vi "NI9252_CREATE_TASK.vi"() -> ()   [LabVIEW 2022 SP3]
uses:
  <vilib>/Analysis/baseanly.llb/Mean (DBL).vi
  <vilib>/express/express shared/transition.llb/Dynamic To Waveform Array.vi
  <vilib>/express/express signal manip/GetorSetDDTAttributes/Set DDT Attributes/SetT0.vi
  <vilib>/express/express signal manip/GetorSetDDTAttributes/Set DDT Attributes/sub Set StartTimeStamp.vi
  <vilib>/express/express shared/transition.llb/Waveform Array To Dynamic.vi
  <vilib>/express/express signal manip/GetorSetDDTAttributes/Set DDT Attributes/Set DDT Properties.xnode
  <vilib>/Analysis/NI_AALBase.lvlib
  <vilib>/express/express signal manip/GetorSetDDTAttributes/Set DDT Attributes/Set DDT Attributes.lvlib
panel:
  in  "Enable":bool=TRUE
  in  "number of samples":i32=60
  in  "rate":dbl=60.0
  out "Waveform Graph 2":dbl[](graph)
  out "Waveform Graph":dbl[](graph)
  out "Waveform Chart 2":dynamicdata(graph)
  out "Waveform Chart":dynamicdata(graph)
  out "Saving Data":bool
  out "Filename Out":path
  in  "Filename":path=path "C:/1. Rocket Research Project/CollectedData/Test_Firing/Constant Chamber Pressure/DataFileThrustWooden.lvm"
  in  "Signal Index 2":i32
  in  "Signal Index":i32
  in  "stop":bool
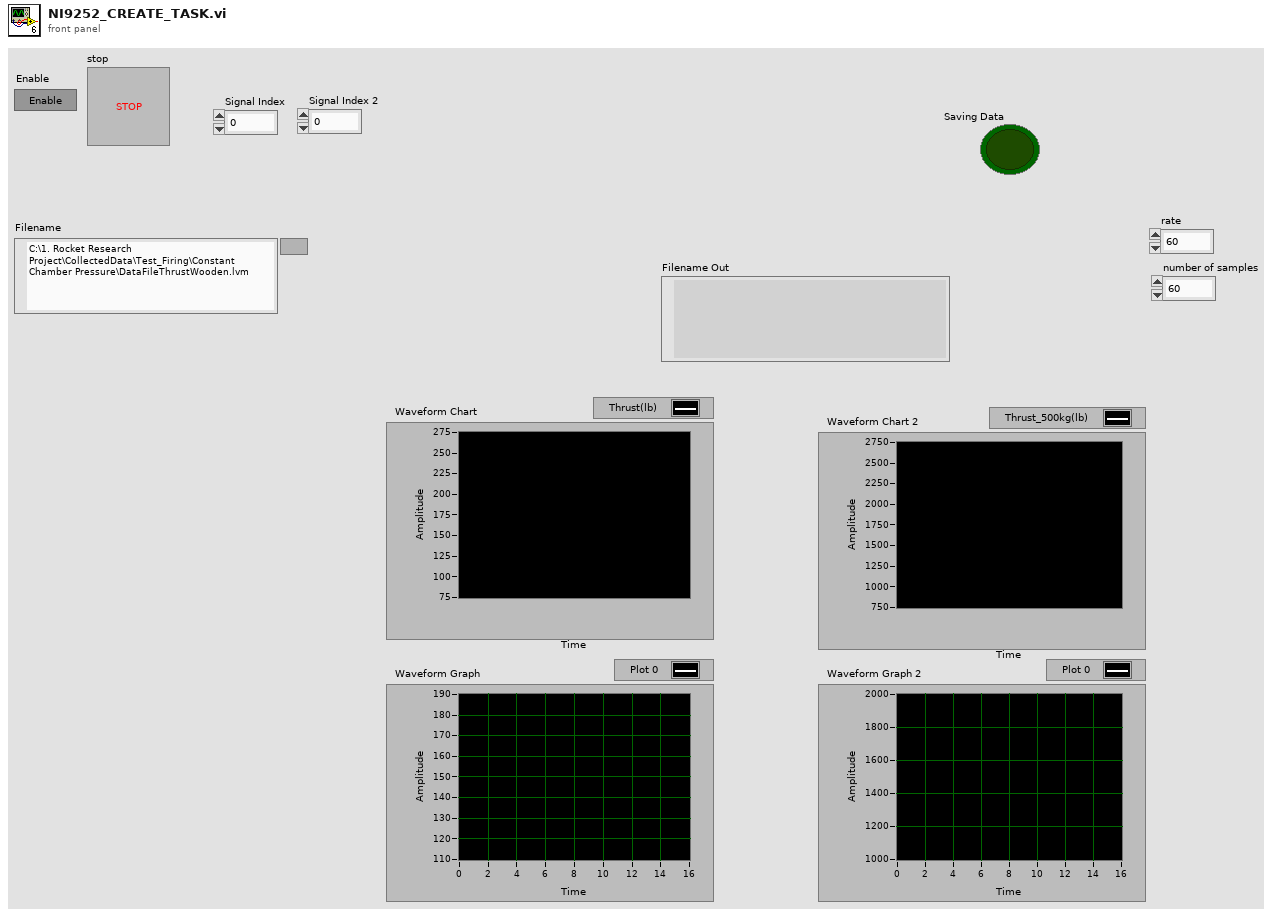
[diagram p1: front panel]
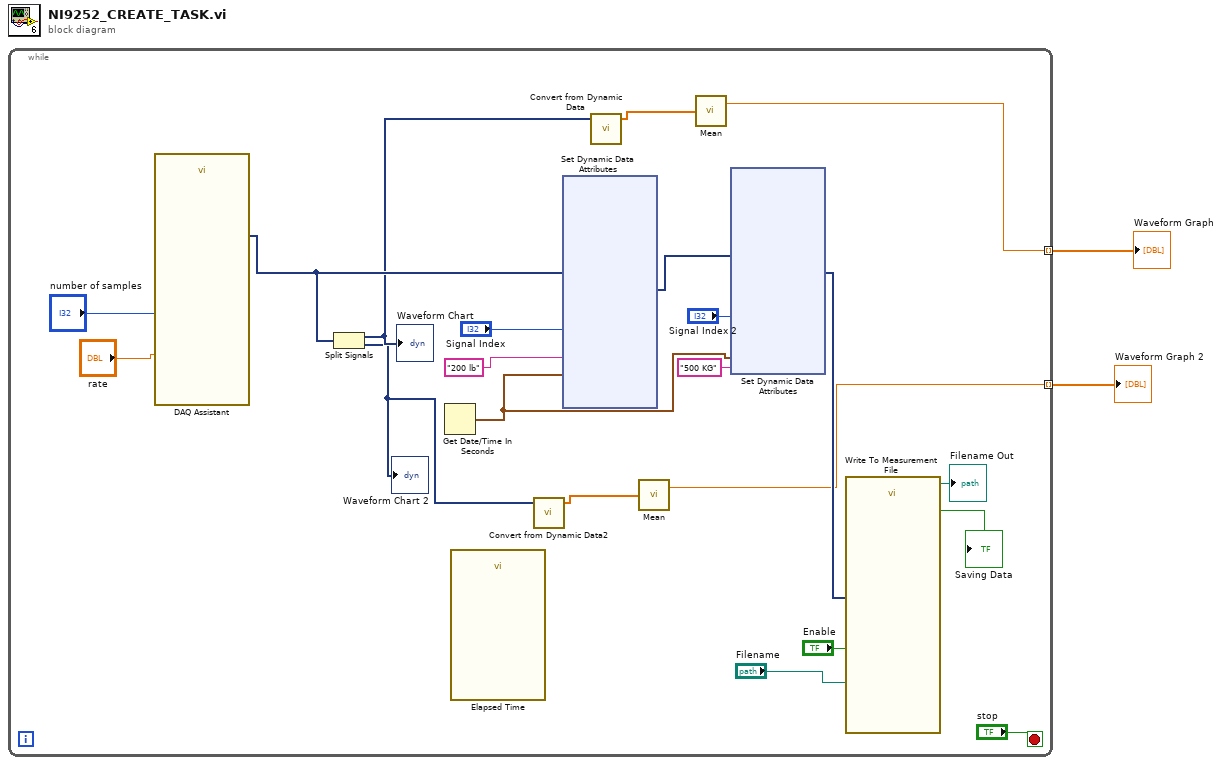
[diagram p0: block diagram]
diagram:
  n1 = while {
    tunnel: [w10] -> w2 mode=indexing
    tunnel: [w7] -> w1 mode=indexing
    stop <- "stop" stop-if-true
    n2 = call "DAQ Assistant"("rate"="rate", "number of samples"="number of samples") -> ("data"=w13:dynamicdata)  [unwired: 14 in, 3 out]
    n3 = Split Signals(w13) -> (w12:dynamicdata, w8:dynamicdata)  [unwired: 2 in]
    "Waveform Chart" <- w12
    "Waveform Chart 2" <- w8
    n4 = Get Date/Time In Seconds() -> (seconds since 1Jan1904=w4:timestamp)
    n5 = call "Elapsed Time"() -> ()  [unwired: 12 in, 8 out]
    n6 = call "Convert from Dynamic Data2"("Dynamic Data Type"=w8) -> ("Array"=w9:dbl[])  [unwired: 3 in]
    n7 = xnode "Set Dynamic Data Attributes"("Signals In"=w13, "Signal Index"="Signal Index", "Signal Name"="200 lb", "Start Timestamp"=w4) -> ("Signals Out"=w20:dynamicdata)  [unwired: 2 in, 1 out]
    n8 = call "Convert from Dynamic Data"("Dynamic Data Type"=w12) -> ("Array"=w11:dbl[])  [unwired: 3 in]
    n9 = call-poly <vilib>:"Mean.vi"("X"=w9) -> ("mean"=w7:dbl)  [unwired: 1 out]
    n10 = call-poly <vilib>:"Mean.vi"("X"=w11) -> ("mean"=w10:dbl)  [unwired: 1 out]
    n11 = xnode "Set Dynamic Data Attributes"("Signals In"=w20, "Signal Index"="Signal Index 2", "Signal Name"="500 KG", "Start Timestamp"=w4) -> ("Signals Out"=w17:dynamicdata)  [unwired: 1 in, 1 out]
    n12 = call "Write To Measurement File"("Signals"=w17, "Enable"="Enable", "Filename"="Filename") -> ("Filename Out"=→"Filename Out":path, "Saving Data"=→"Saving Data":bool)  [unwired: 14 in, 1 out]
  }
  "Waveform Graph" <- w2
  "Waveform Graph 2" <- w1
